vi "DesignPatterns_GetNoteTextAndLinks.vi"(11 "ClassText":string="\t\t\t<Links>\n\t\t\t\t<Link id='ToRequest' name='' source='Request'/>\n\t\t\t</Links>\n\t") -> (2 "Links":T1[](array[typedef]), 3 "Text":string)   [LabVIEW 2016]
uses:
  <resource>/Framework/Providers/Open_GDS/UML/DesignPattern/SubVIs/DesignPatterns_NoteLink.ctl
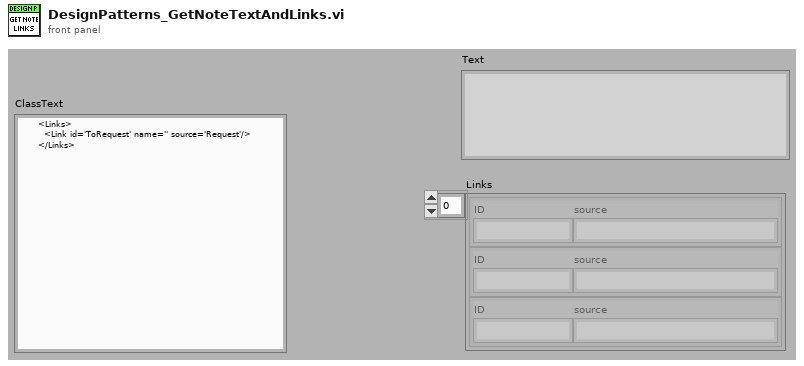
[diagram p1: front panel]
types:
  T1 = typedef "DesignPatterns_NoteLink.ctl" = cluster{"ID":string, "source":string}
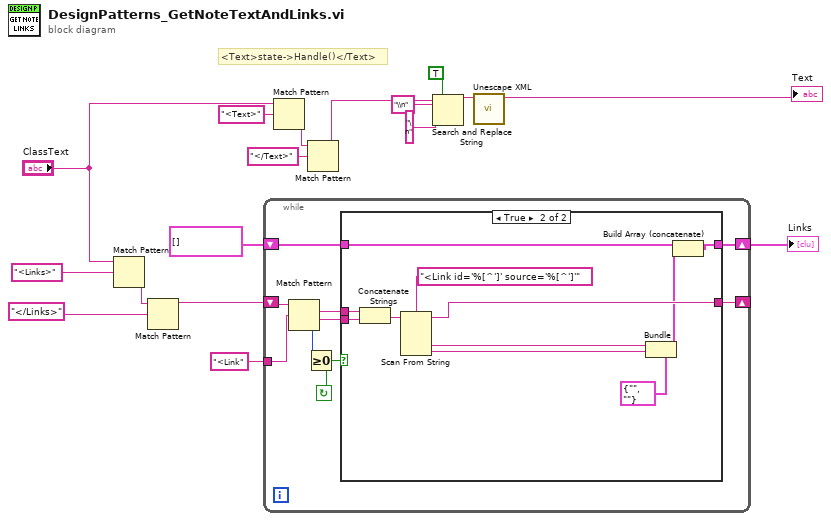
[diagram p0: block diagram]
diagram:
  # "<Text>state->Handle()</Text>"
  n1 = Match Pattern(string="ClassText", regular expression="<Links>") -> (after substring=w16:string)  [unwired: 4 out]
  n2 = Match Pattern(string=w16, regular expression="</Links>") -> (before substring=w14:string)  [unwired: 4 out]
  n3 = while {
    shift-right: [w20] -> _
    shift-left: w14 -> [w24]
    tunnel: "<Link" ("regular expression") -> [w23]
    shift-right: [w18] -> w12
    shift-left: T1[] [] ("Links") -> [w19]
    stop <- w21 continue-if-true
    n4 = Match Pattern(string=w24, regular expression=w23) -> (match substring=w25:string, after substring=w26:string, offset past match=w22:i32)  [unwired: 2 out]
    n5 = Greater Or Equal To 0?(x=w22) -> (x >= 0?=w21:bool)
    n6 = case shown="True" w21 {
      tunnel: w26 -> [_ w37]
      tunnel: w25 -> [_ w36]
      tunnel: [_ w35] -> w20
      tunnel: w19 -> [w27 w33]
      tunnel: [w27 w32] -> w18
      frame False {
      }
      frame True {
        n7 = Concatenate Strings(w36, w37) -> (w38:string)
        n8 = Scan From String(format string="<Link id='%[^']' source='%[^']'", input string=w38) -> (remaining string=w35:string, output 1=w31:string, output 2=w29:string)  [unwired: 2 in, 4 out]
        n9 = Bundle(cluster=T1 {"ID"="", "source"=""}, "ID"=w31, "source"=w29) -> (w30:T1)
        n10 = Build Array (concatenate)(w33, w30) -> (w32:T1[])
      }
    }
  }
  "Links" <- w12
  n11 = Match Pattern(string="ClassText", regular expression="<Text>") -> (after substring=w10:string)  [unwired: 4 out]
  n12 = Match Pattern(string=w10, regular expression="</Text>") -> (before substring=w2:string)  [unwired: 4 out]
  n13 = Search and Replace String(replace all?=TRUE ("replace all? (F)"), input string=w2, search string="\\n", replace string="\n" ("replace string (\"\")")) -> (result string=w3:string)  [unwired: 1 in, 6 out]
  n14 = call <vilib>:"Unescape XML.vi"("XML String In"=w3) -> ("XML String Out"=→"Text":string)  [unwired: 1 in, 9 out]
